vi "AES - Encrypt String.vi"(8 "error in (no error)":errorcluster, 9 "IV":u8[](array[numeric]), 10 "key":u8[](array[numeric]), 11 "string to encrypt":string) -> (0 "error out":errorcluster, 3 "encrypted string":string)   [LabVIEW 2013]
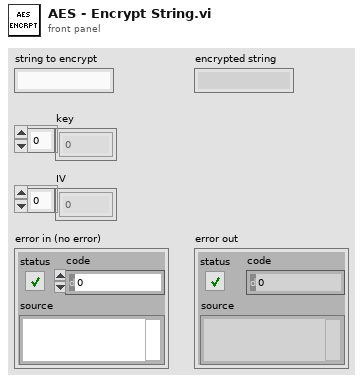
[diagram p1: front panel]
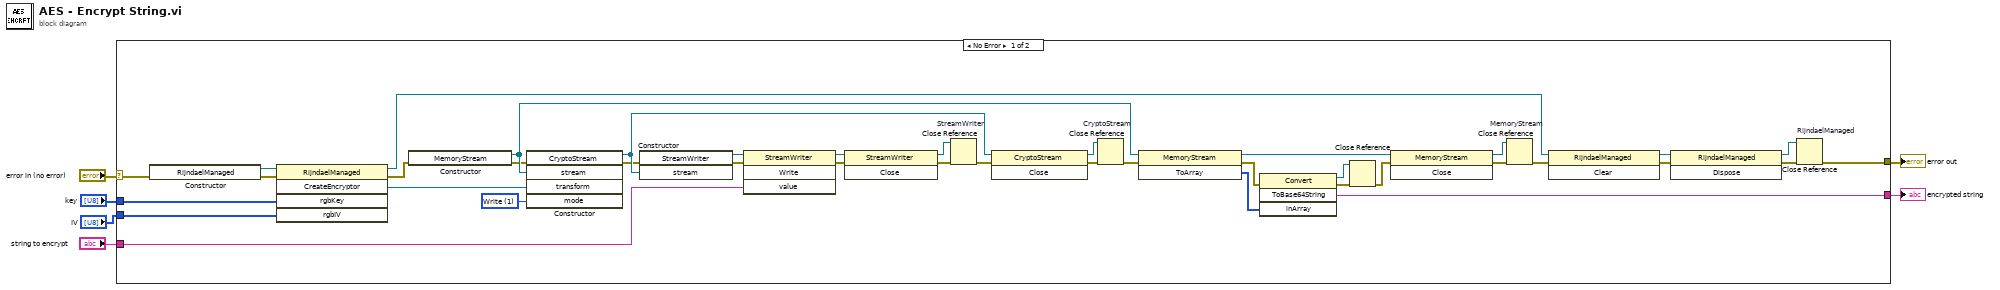
[diagram p0: block diagram]
diagram:
  n1 = case shown="No Error" "error in (no error)" {
    selector: "error in (no error)" -> [w16 w46]
    tunnel: "IV" -> [w26 _]
    tunnel: "key" -> [w25 _]
    tunnel: [w15 w46] -> w3
    tunnel: "string to encrypt" -> [w11 _]
    tunnel: [w13 _] -> w1
    frame No Error {
      w19 = 1 items=["Read", "Write"] ("mode")
      n2 = constructor class="RijndaelManaged"(error in=w16) -> (reference out=w21:refnum<k24>, error out=w20:errorcluster)  [unwired: 2 in, 1 out]
      n3 = invoke class="RijndaelManaged" method="CreateEncryptor"(reference=w21, error in=w20, "rgbKey"=w25, "rgbIV"=w26) -> (reference out=w40:refnum<k24>, error out=w22:errorcluster, "CreateEncryptor"=w18:refnum<k24>)  [unwired: 1 in, 2 out]
      n4 = constructor class="MemoryStream"(error in=w22) -> (reference out=w31:refnum<k24>, error out=w17:errorcluster)  [unwired: 2 in, 1 out]
      n5 = constructor class="CryptoStream"(error in=w17, "stream"=w31, "transform"=w18, "mode"=w19) -> (reference out=w29:refnum<k24>, error out=w23:errorcluster)  [unwired: 2 in, 4 out]
      n6 = constructor class="StreamWriter"(error in=w23, "stream"=w29) -> (reference out=w24:refnum<k24>, error out=w12:errorcluster)  [unwired: 2 in, 2 out]
      n7 = invoke class="StreamWriter" method="Write"(reference=w24, error in=w12, "value"=w11) -> (reference out=w27:refnum<k24>, error out=w28:errorcluster)  [unwired: 1 in, 2 out]
      n8 = invoke class="StreamWriter" method="Close"(reference=w27, error in=w28) -> (reference out=w33:refnum<k24>, error out=w30:errorcluster)  [unwired: 1 in, 1 out]
      n9 = Close Reference "StreamWriter"(reference=w33, error in (no error)=w30) -> (error out=w32:errorcluster)
      n10 = invoke class="CryptoStream" method="Close"(reference=w29, error in=w32) -> (reference out=w35:refnum<k24>, error out=w34:errorcluster)  [unwired: 1 in, 1 out]
      n11 = Close Reference "CryptoStream"(reference=w35, error in (no error)=w34) -> (error out=w36:errorcluster)
      n12 = invoke class="MemoryStream" method="ToArray"(reference=w31, error in=w36) -> (reference out=w37:refnum<k24>, error out=w10:errorcluster, "ToArray"=w14:u8[])  [unwired: 1 in]
      n13 = invoke class="Convert" method="ToBase64String"(error in=w10, "inArray"=w14) -> (reference out=w8:refnum<k24>, error out=w9:errorcluster, "ToBase64String"=w13:string)  [unwired: 2 in, 1 out]
      n14 = Close Reference(reference=w8, error in (no error)=w9) -> (error out=w7:errorcluster)
      n15 = invoke class="MemoryStream" method="Close"(reference=w37, error in=w7) -> (reference out=w39:refnum<k24>, error out=w38:errorcluster)  [unwired: 1 in, 1 out]
      n16 = Close Reference "MemoryStream"(reference=w39, error in (no error)=w38) -> (error out=w43:errorcluster)
      n17 = invoke class="RijndaelManaged" method="Clear"(reference=w40, error in=w43) -> (reference out=w42:refnum<k24>, error out=w41:errorcluster)  [unwired: 1 in, 1 out]
      n18 = invoke class="RijndaelManaged" method="Dispose"(reference=w42, error in=w41) -> (reference out=w45:refnum<k24>, error out=w44:errorcluster)  [unwired: 1 in, 1 out]
      n19 = Close Reference "RijndaelManaged"(reference=w45, error in (no error)=w44) -> (error out=w15:errorcluster)
    }
    frame Error {
    }
  }
  "error out" <- w3
  "encrypted string" <- w1
